vi "Get XML Attributes.vi"(8 "error in (no error)":errorcluster, 11 "Element Array in":refnum<class "Element Array.lvclass">) -> (0 "error out":errorcluster, 2 "XML Attributes":cluster{"Name":string, "Value":string}[](array[cluster]), 3 "Element Array out":refnum<class "Element Array.lvclass">)   [LabVIEW 2023, in "VILab.lvlib" / "Element Array.lvclass"]
uses:
  Element Array.lvclass
  Element Array.lvclass/Element Array.ctl
  Data Item/Data Item.lvclass
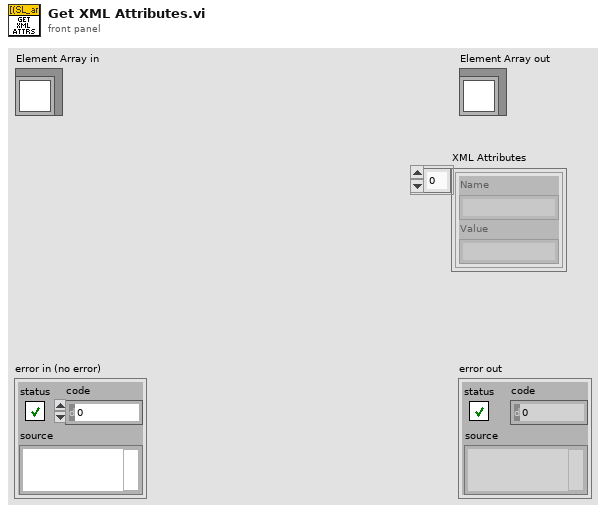
[diagram p1: front panel]
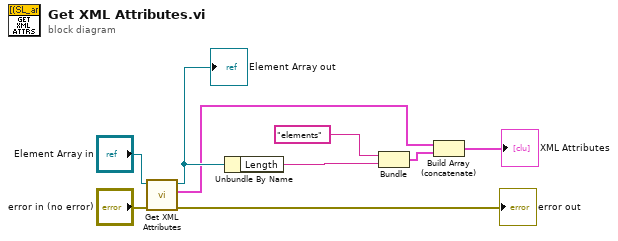
[diagram p0: block diagram]
diagram:
  n1 = call-parent "Get XML Attributes.vi"("error in (no error)"="error in (no error)", "Data Item in"="Element Array in") -> ("error out"=→"error out":errorcluster, "XML Attributes"=w3:cluster{"Name":string, "Value":string}[], "Data Item out"=w4:refnum<class "Element Array.lvclass">)  [unwired: 7 in]
  "Element Array out" <- w4
  n2 = Unbundle By Name(w4) -> ("Length"=w5:string)
  n3 = Bundle("elements", "Length"=w5) -> (w2:cluster{string, "Length":string})  [unwired: 1 in]
  n4 = Build Array (concatenate)(w3, w2) -> (→"XML Attributes":cluster{"Name":string, "Length":string}[])
